vi "Finish.vi"   [LabVIEW 2012]
doc: "This VI is called just before exiting. It is expected to close I/O refnum, save collected data, etc."
uses:
  <vilib>/Rock Robotics/WPI/Joystick/WPI_JoystickGetSetRefNum.vi
types:
  T1 = typedef "WPI_DigitalInputDevRef.ctl" = cluster{"DevStatus":errorcluster, "DIO Channel":T2, "Digital Module":T3}
  T2 = typedef "FPGA_DIOChannel.ctl" = enum8{"DIO 1", "DIO 2", "DIO 3", "DIO 4", "DIO 5", "DIO 6", "DIO 7", "DIO 8", "DIO 9", "DIO 10", "DIO 11", "DIO 12", "DIO 13", "DIO 14", "Invalid"}
  T3 = typedef "FPGA_TypedefDigitalModule.ctl" = enum16{"Digital Module 1", "Digital Module 2"}
  T4 = typedef "WPI_CounterDevRef.ctl" = cluster{"DevStatus":errorcluster, "CntIndex":T5}
  T5 = typedef "FPGA_CounterCtrSystemIndex.ctl" = enum8{"Ctr 0", "Ctr 1", "Ctr 2", "Ctr 3", "Ctr 4", "Ctr 5", "Ctr 6", "Ctr 7", "Invalid"}
  T6 = typedef "WPI_JoystickDevRef.ctl" = cluster{"Device":T7}
  T7 = typedef "WPI_JoystickDeviceEnum.ctl" = enum16{"USB 1", "USB 2", "USB 3", "USB 4", "Kinect 1", "Kinect 2"}
  T8 = typedef "WPI_CameraDevRef.ctl" = cluster{"Camera Address":string, "CameraStatus":errorcluster, "Acquire Image Notifier":refnum<notifier>}
  T9 = typedef "WPI_I2CDevRef.ctl" = cluster{"DevStatus":errorcluster, "Digital Module":T3, "Device Address":u8}
  T10 = typedef "WPI_GyroDevRef.ctl" = cluster{"DevStatus":errorcluster, "Analog Module":T11, "Analog Channel":T12, "Offset":dbl, "Gain (VoltsPerDegree/Second)":dbl}
  T11 = typedef "FPGA_TypedefAnalogModule.ctl" = enum16{"Analog Module 1", "Analog Module 2"}
  T12 = typedef "FPGA_AIChannel.ctl" = enum8{"AI 1", "AI 2", "AI 3", "AI 4", "AI 5", "AI 6", "AI 7", "AI 8", "Invalid"}
  T13 = typedef "WPI_AnalogChannelDevRef.ctl" = cluster{"DevStatus":errorcluster, "Analog Module":T11, "Analog Channel":T12}
  T14 = typedef "WPI_MotorControlDeviceRef.ctl" = cluster{"DeviceStatus":errorcluster, "Type":enum16{"PWM", "CAN"}, "PWM":cluster{"Digital Module":T3, "PWM Channel":T15, "DeadBand":T16}, "CAN":cluster{"Device Number":u8, "Control Mode":T17, "Semaphore":T18, "Max Vout":dbl}, "Invert":bool, "TransformRef":T19, "InvTransformRef":T19}
  T15 = typedef "FPGA_DIOPWMChannel.ctl" = enum8{"PWM 1", "PWM 2", "PWM 3", "PWM 4", "PWM 5", "PWM 6", "PWM 7", "PWM 8", "PWM 9", "PWM 10", "Invalid"}
  T16 = typedef "WPI_PWMDeadband.ctl" = cluster{"Name":string, "maxPositivePwm":i32, "minPositivePwm":i32, "centerPwm":i32, "maxNegativePwm":i32, "minNegativePwm":i32, "angularRange":u16}
  T17 = typedef "WPI_CANJaguar_ControlMode.ctl" = enum8{"Percent VBus", "Current", "Speed", "Position", "Voltage"}
  T18 = typedef "Semaphore RefNum" = refnum<k1>
  T19 = typedef "WPI_PWMTransform_ConPane.ctl" = refnum<vi>
  T20 = typedef "WPI_EncoderDevRef.ctl" = cluster{"DevStatus":errorcluster, "EncoderIndex":T21, "CounterIndex":T5, "DistancePerCount":dbl, "Decoding Type":T22}
  T21 = typedef "FPGA_EncoderIdx.ctl" = enum8{"Enc 0", "Enc 1", "Enc 2", "Enc 3", "Invalid"}
  T22 = typedef "WPI_EncoderType.ctl" = enum16{"1x", "2x", "4x"}
  T23 = typedef "WPI_SolenoidDevRef.ctl" = cluster{"DevStatus":errorcluster, "Solenoid Module":T24, "Forward Solenoid Channel":T25, "Reverse Solenoid Channel":T25}
  T24 = typedef "FPGA_TypedefSolenoidModule.ctl" = enum16{"Solenoid Module 1", "Solenoid Module 2"}
  T25 = typedef "WPI_SolenoidChannel.ctl" = enum8{"Solenoid 1", "Solenoid 2", "Solenoid 3", "Solenoid 4", "Solenoid 5", "Solenoid 6", "Solenoid 7", "Solenoid 8", "Invalid"}
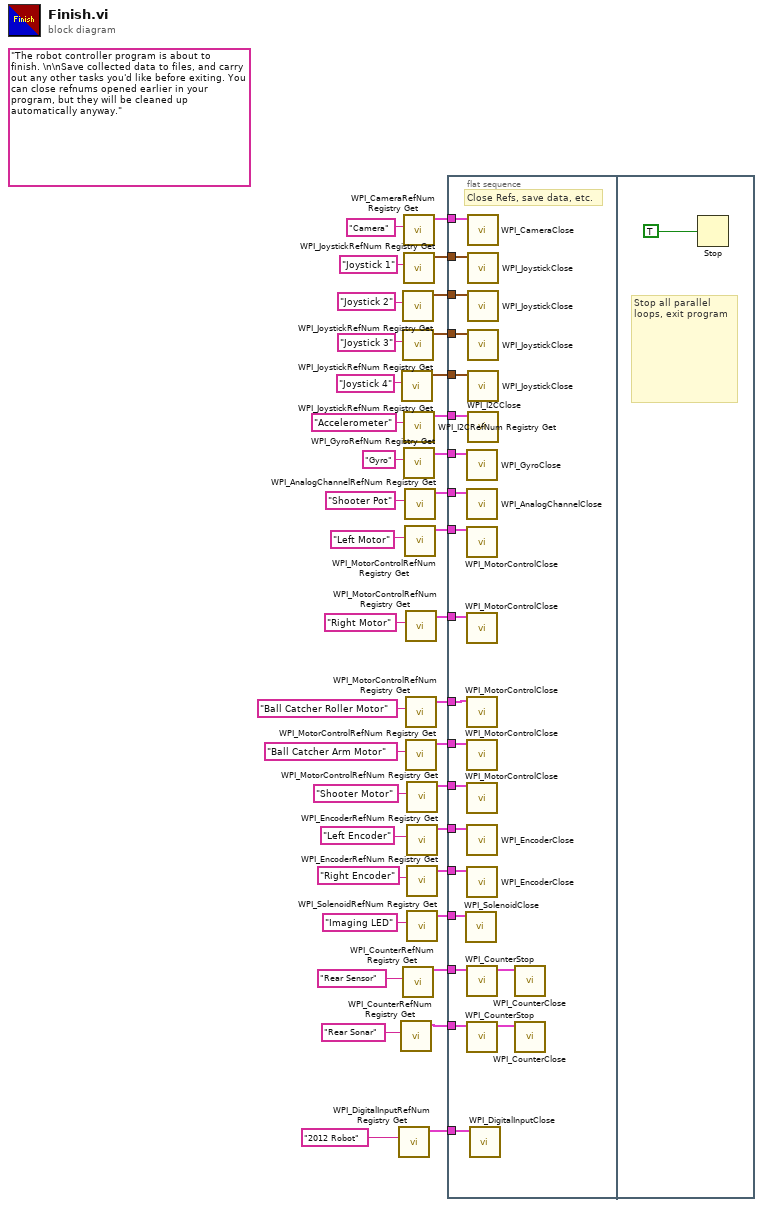
[diagram p0: block diagram]
diagram:
  (unwired) "The robot controller program is about to finish. \n\nSave collected data to files, and carry out any other tasks you'd like before exiting. You can close refnums opened earlier in your program, but they will be cleaned up automatically anyway."
  n1 = call <vilib>:"WPI_DigitalInputRefNum Registry Get.vi"("refnum name"="2012 Robot") -> ("DigitalInputDevRef"=w3:T1)  [unwired: 9 in, 1 out]
  n2 = call <vilib>:"WPI_CounterRefNum Registry Get.vi"("refnum name"="Rear Sonar") -> ("CounterDevRef"=w6:T4)  [unwired: 9 in, 1 out]
  n3 = call <vilib>:"WPI_JoystickRefNum Registry Get.vi"("refnum name"="Joystick 4") -> ("JoystickDevRef"=w13:T6)  [unwired: 1 in, 9 out]
  n4 = call <vilib>:"WPI_JoystickRefNum Registry Get.vi"("refnum name"="Joystick 2") -> ("JoystickDevRef"=w37:T6)  [unwired: 1 in, 9 out]
  n5 = call <vilib>:"WPI_JoystickRefNum Registry Get.vi"("refnum name"="Joystick 3") -> ("JoystickDevRef"=w15:T6)  [unwired: 1 in, 9 out]
  n6 = call <vilib>:"WPI_CounterRefNum Registry Get.vi"("refnum name"="Rear Sensor") -> ("CounterDevRef"=w5:T4)  [unwired: 9 in, 1 out]
  n7 = call <vilib>:"WPI_CameraRefNum Registry Get.vi"("refnum name"="Camera") -> ("CameraDevRef"=w36:T8)  [unwired: 1 in, 9 out]
  n8 = call <vilib>:"WPI_JoystickRefNum Registry Get.vi"("refnum name"="Joystick 1") -> ("JoystickDevRef"=w24:T6)  [unwired: 9 in, 1 out]
  n9 = call <vilib>:"WPI_I2CRefNum Registry Get.vi"("refnum name"="Accelerometer") -> ("I2CDevRef"=w23:T9)  [unwired: 9 in, 1 out]
  n10 = call <vilib>:"WPI_GyroRefNum Registry Get.vi"("refnum name"="Gyro") -> ("GyroDevRef"=w25:T10)  [unwired: 9 in, 1 out]
  n11 = call <vilib>:"WPI_AnalogChannelRefNum Registry Get.vi"("refnum name"="Shooter Pot") -> ("AIDeviceRef"=w18:T13)  [unwired: 9 in, 1 out]
  n12 = call <vilib>:"WPI_MotorControlRefNum Registry Get.vi"("refnum name"="Left Motor") -> ("MotorControlDevRef"=w26:T14)  [unwired: 9 in, 1 out]
  n13 = call <vilib>:"WPI_MotorControlRefNum Registry Get.vi"("refnum name"="Right Motor") -> ("MotorControlDevRef"=w27:T14)  [unwired: 9 in, 1 out]
  n14 = call <vilib>:"WPI_MotorControlRefNum Registry Get.vi"("refnum name"="Ball Catcher Roller Motor") -> ("MotorControlDevRef"=w9:T14)  [unwired: 9 in, 1 out]
  n15 = call <vilib>:"WPI_MotorControlRefNum Registry Get.vi"("refnum name"="Ball Catcher Arm Motor") -> ("MotorControlDevRef"=w10:T14)  [unwired: 9 in, 1 out]
  n16 = call <vilib>:"WPI_MotorControlRefNum Registry Get.vi"("refnum name"="Shooter Motor") -> ("MotorControlDevRef"=w21:T14)  [unwired: 9 in, 1 out]
  n17 = call <vilib>:"WPI_EncoderRefNum Registry Get.vi"("refnum name"="Left Encoder") -> ("EncoderDevRef"=w28:T20)  [unwired: 9 in, 1 out]
  n18 = call <vilib>:"WPI_EncoderRefNum Registry Get.vi"("refnum name"="Right Encoder") -> ("EncoderDevRef"=w29:T20)  [unwired: 9 in, 1 out]
  n19 = call <vilib>:"WPI_SolenoidRefNum Registry Get.vi"("refnum name"="Imaging LED") -> ("SolenoidDevRef"=w1:T23)  [unwired: 9 in, 1 out]
  n20 = flat-sequence {
    tunnel: w37 -> [w59]
    tunnel: w36 -> [w58]
    tunnel: w29 -> [w57]
    tunnel: w28 -> [w56]
    tunnel: w27 -> [w55]
    tunnel: w26 -> [w54]
    tunnel: w25 -> [w53]
    tunnel: w24 -> [w52]
    tunnel: w23 -> [w51]
    tunnel: w21 -> [w50]
    tunnel: w18 -> [w49]
    tunnel: w15 -> [w48]
    tunnel: w13 -> [w47]
    tunnel: w10 -> [w46]
    tunnel: w9 -> [w45]
    tunnel: w6 -> [w42]
    tunnel: w5 -> [w41]
    tunnel: w3 -> [w40]
    tunnel: w1 -> [w39]
    frame #0 {
      # "Close Refs, save data, etc."
      n21 = call <vilib>:"WPI_SolenoidClose.vi"("SolenoidDevRef"=w39) -> ()  [unwired: 10 in, 1 out]
      n22 = call <vilib>:"WPI_GyroClose.vi"("GyroDevRef"=w53) -> ()  [unwired: 1 in, 10 out]
      n23 = call <vilib>:"WPI_AnalogChannelClose.vi"("AIDeviceRef"=w49) -> ()  [unwired: 10 in, 1 out]
      n24 = call <vilib>:"WPI_MotorControlClose.vi"("MotorControlDevRef"=w54) -> ()  [unwired: 1 in, 10 out]
      n25 = call <vilib>:"WPI_MotorControlClose.vi"("MotorControlDevRef"=w55) -> ()  [unwired: 1 in, 10 out]
      n26 = call <vilib>:"WPI_MotorControlClose.vi"("MotorControlDevRef"=w45) -> ()  [unwired: 1 in, 10 out]
      n27 = call <vilib>:"WPI_MotorControlClose.vi"("MotorControlDevRef"=w46) -> ()  [unwired: 1 in, 10 out]
      n28 = call <vilib>:"WPI_MotorControlClose.vi"("MotorControlDevRef"=w50) -> ()  [unwired: 1 in, 10 out]
      n29 = call <vilib>:"WPI_EncoderClose.vi"("EncoderDevRef"=w56) -> ()  [unwired: 2 in, 9 out]
      n30 = call <vilib>:"WPI_EncoderClose.vi"("EncoderDevRef"=w57) -> ()  [unwired: 2 in, 9 out]
      n31 = call <vilib>:"WPI_CounterStop.vi"("CounterDevRef in"=w41) -> ("CounterDevRef out"=w44:T4)  [unwired: 9 in, 1 out]
      n32 = call <vilib>:"WPI_CounterStop.vi"("CounterDevRef in"=w42) -> ("CounterDevRef out"=w43:T4)  [unwired: 9 in, 1 out]
      n33 = call <vilib>:"WPI_CameraClose.vi"("CameraDevRef"=w58) -> ()  [unwired: 1 in, 10 out]
      n34 = call <vilib>:"WPI_JoystickClose.vi"("JoystickDevRef"=w52) -> ()  [unwired: 11 in]
      n35 = call <vilib>:"WPI_JoystickClose.vi"("JoystickDevRef"=w59) -> ()  [unwired: 11 out]
      n36 = call <vilib>:"WPI_JoystickClose.vi"("JoystickDevRef"=w48) -> ()  [unwired: 11 out]
      n37 = call <vilib>:"WPI_JoystickClose.vi"("JoystickDevRef"=w47) -> ()  [unwired: 11 out]
      n38 = call <vilib>:"WPI_I2CClose.vi"("I2CDevRef"=w51) -> ()  [unwired: 1 in, 10 out]
      n39 = call <vilib>:"WPI_DigitalInputClose.vi"("DigitalInputDevRef"=w40) -> ()  [unwired: 10 in, 1 out]
      n40 = call <vilib>:"WPI_CounterClose.vi"("CounterDevRef"=w44) -> ()  [unwired: 10 in, 1 out]
      n41 = call <vilib>:"WPI_CounterClose.vi"("CounterDevRef"=w43) -> ()  [unwired: 10 in, 1 out]
    }
    frame #1 {
      # "Stop all parallel\nloops, exit program"
      n42 = Stop(stop? (T)=TRUE ("Quit")) -> ()
    }
  }
